vi "Odbior danych z PC 2.vi"(8 "error in (no error)":errorcluster, 11 "connection ID":refnum<k16>) -> (0 "error out":errorcluster, 1 "output cluster":T2 {"Cluster"."array of cans"."type" items=["CAN Data", "CAN Remote"]; "Cluster"."array of cans"."identifier" format="%.0x"}, 2 "konf":T1 {"type" items=["CAN Data", "CAN Remote"]; "identifier" format="%.0x"}, 3 "connection ID out":refnum<k16>)   [LabVIEW 2015]
uses:
  <vilib>/RioEmbeddedCAN/RioEmbeddedCAN.llb/CANFrameControl.ctl
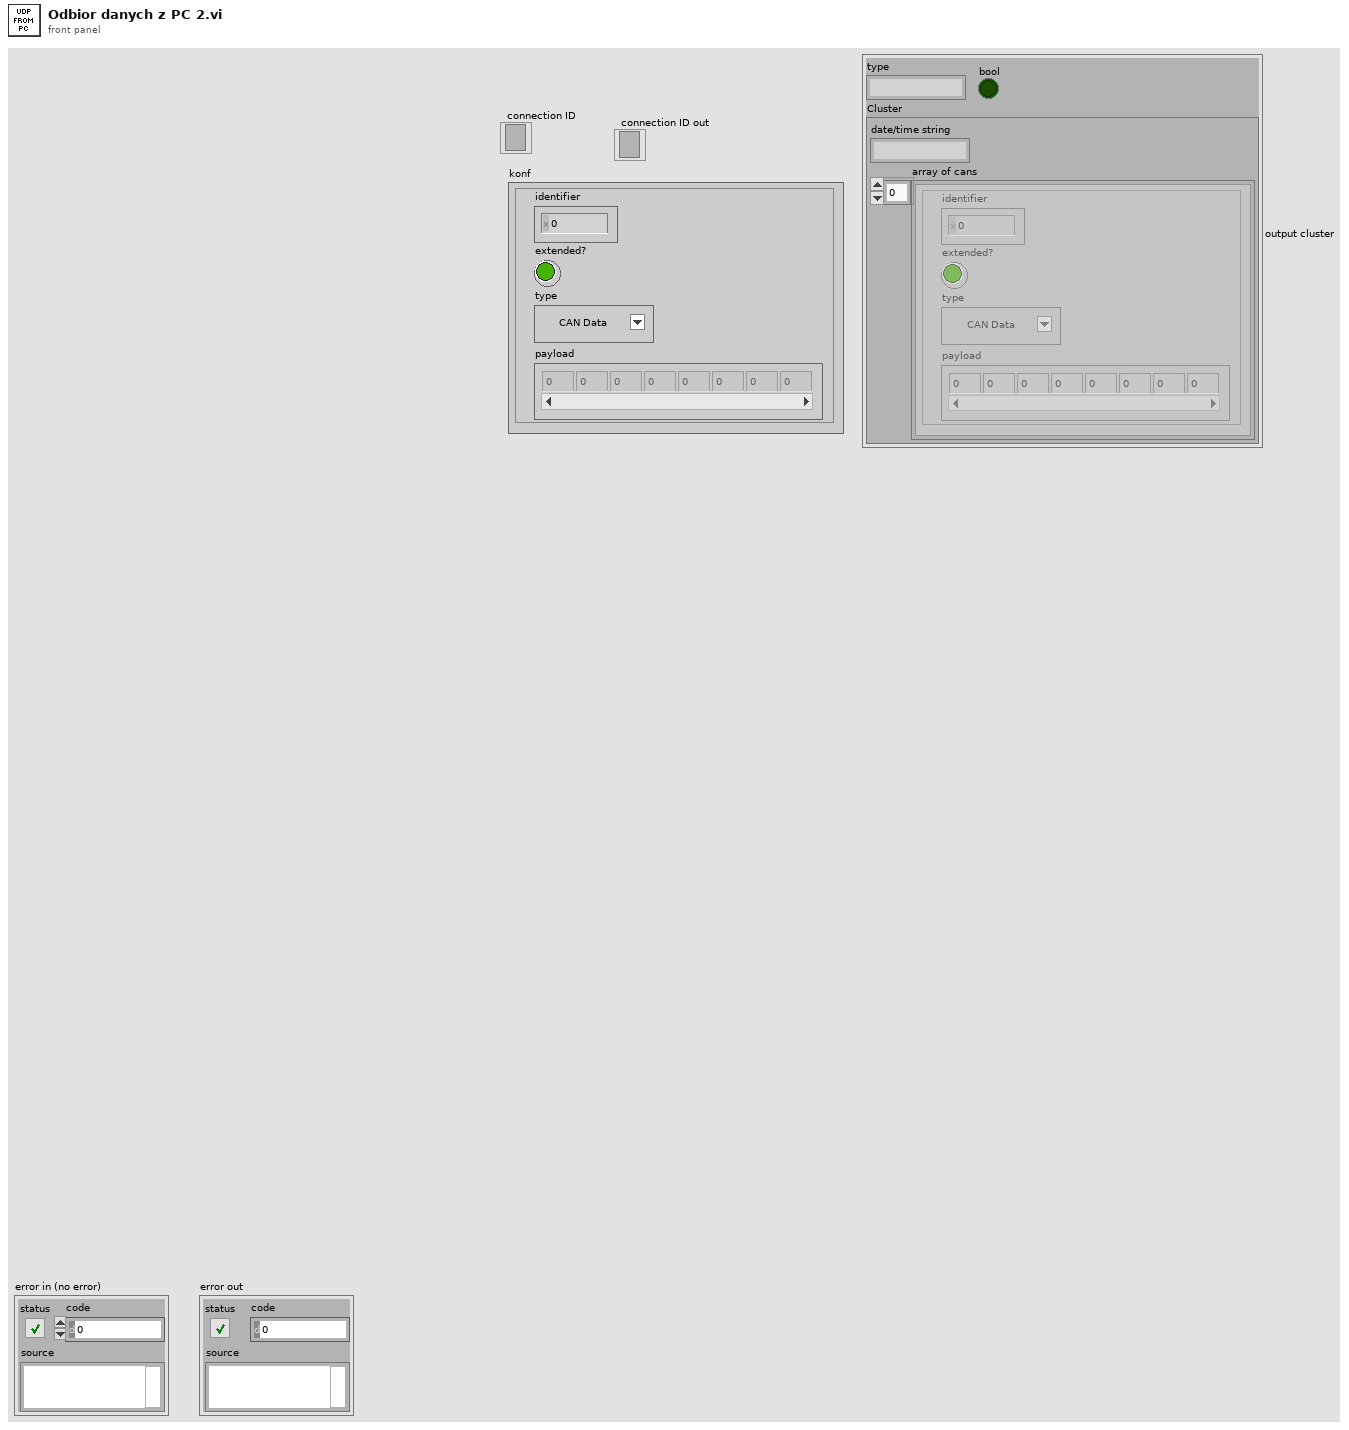
[diagram p1: front panel]
types:
  T1 = typedef "CANFrameControl.ctl" = cluster{"identifier":u32, "extended?":bool, "type":u8, "payload":u8[]}
  T2 = cluster{"type":string, "Cluster":cluster{"date/time string":string, "array of cans":T1[]}, "bool":bool}
  T3 = cluster{"date/time string":string, "array of cans":T1[]}
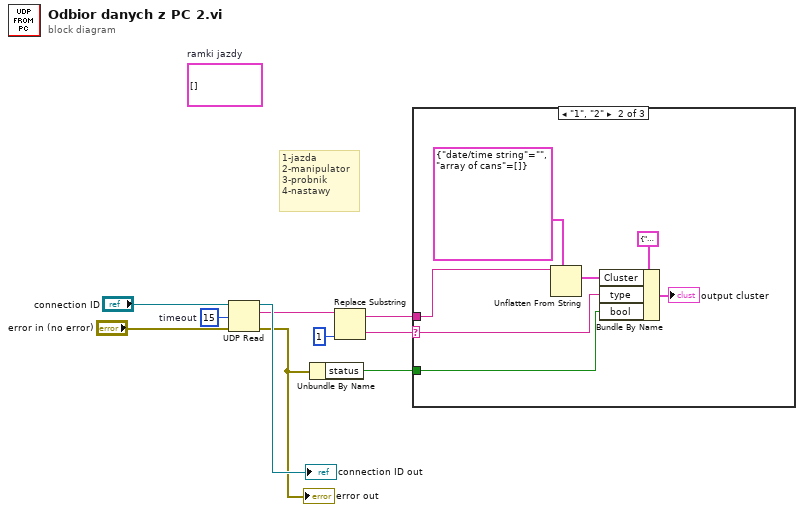
[diagram p0: block diagram]
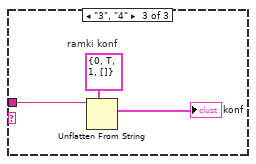
[diagram p3: hidden frame]
diagram:
  w8 = 15  # timeout
  (unwired) T1[] []  # ramki jazdy
  # "1-jazda\n2-manipulator\n3-probnik\n4-nastawy"
  n1 = UDP Read(connection ID="connection ID", timeout ms (25000)=w8, 8:"error in (no error)") -> (data out=w5:string, error out=w2:errorcluster, 3:→"connection ID out":refnum<k16>)  [unwired: 1 in, 2 out]
  "error out" <- w2
  n2 = Unbundle By Name(w2) -> ("status"=w1:bool)
  n3 = Replace Substring(2:1 ("length (len. of substring)"), 5:w5) -> (0:w4:string, 1:w3:string)  [unwired: 2 in]
  n4 = case shown="\"1\", \"2\"" w4 {
    selector: w4 -> [_ w15 _]
    tunnel: w3 -> [_ w16 w18]
    tunnel: w1 -> [_ w12 _]
    frame "False", Default {
    }
    frame "1", "2" {
      n5 = Unflatten From String(type=T3 {"date/time string"="", "array of cans"=[]} ("output cluster"), binary string=w16) -> (value=w14:T3)  [unwired: 3 in, 2 out]
      n6 = Bundle By Name(cluster=T2 {"type"="", "Cluster"={"date/time string"="", "array of cans"=[]}, "bool"=TRUE} ("jazda"), "Cluster"=w14, "type"=w15, "bool"=w12) -> (→"output cluster":T2)
    }
    frame "3", "4" {
      w19 = T1 {"identifier"=0, "extended?"=TRUE, "type"=1, "payload"=[]}  # ramki konf
      n7 = Unflatten From String(type=w19, binary string=w18) -> (value=→"konf":T1)  [unwired: 3 in, 2 out]
    }
  }
